vi "RetrieveDefaultRectangleData.vi"(8 "error in (no error)":errorcluster, 10 "Path":path, 11 "Setting Database In":refnum<class "Setting Database.lvclass">) -> (0 "error out":errorcluster, 2 "Rectangle Settings.lvclass":refnum<class "Rectangle Settings.lvclass">, 3 "Setting Database Out":refnum<class "Setting Database.lvclass">)   [LabVIEW 2019, in "Setting Database.lvclass"]
uses:
  Setting Database.lvclass
  Rectangle Settings/Rectangle Settings.lvclass
  Setting Database.lvclass/Setting Database.ctl
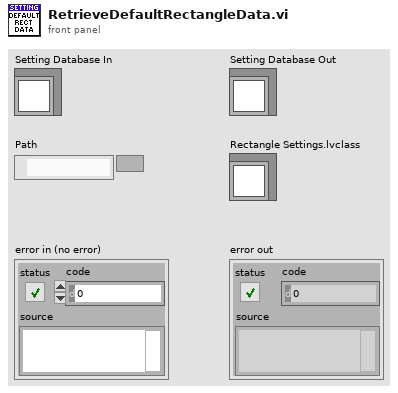
[diagram p1: front panel]
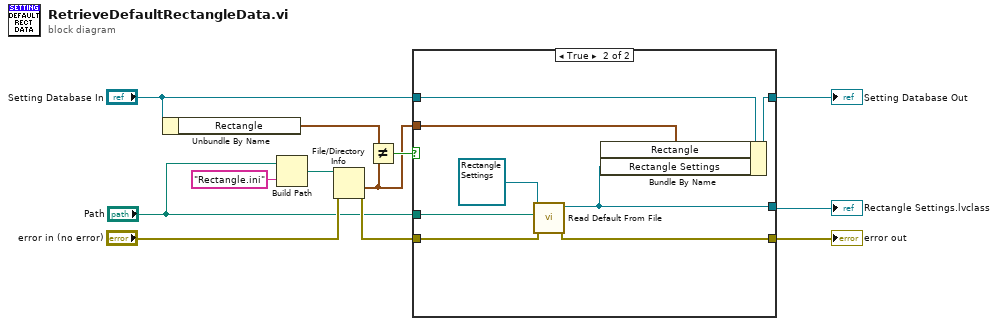
[diagram p0: block diagram]
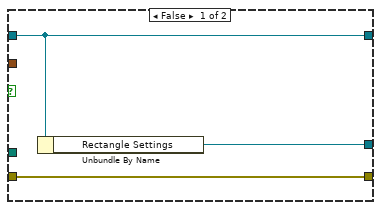
[diagram p2: hidden frame]
diagram:
  n1 = Unbundle By Name("Setting Database In") -> ("Rectangle"=w2:timestamp)
  n2 = Build Path(base path="Path", name or relative path="Rectangle.ini") -> (appended path=w9:path)
  n3 = File/Directory Info(path=w9, error in="error in (no error)") -> (last mod=w1:timestamp, error out=w6:errorcluster)  [unwired: 5 out]
  n4 = Not Equal?(x=w2, y=w1) -> (x != y?=w3:bool)
  n5 = case shown="True" w3 {
    tunnel: [w15 w19] -> w11
    tunnel: "Setting Database In" -> [w14 w22]
    tunnel: [w14 w23] -> w10
    tunnel: w6 -> [w13 w20]
    tunnel: [w13 w21] -> w12
    tunnel: "Path" -> [_ w17]
    tunnel: w1 -> [_ w16]
    frame False {
      n6 = Unbundle By Name(w14) -> ("Rectangle Settings"=w15:refnum<class "Rectangle Settings.lvclass">)
    }
    frame True {
      n7 = call-dynamic "Read Default From File.vi"("error in (no error)"=w20, "Path"=w17, "Rectangle Settings in"=refnum<class "Rectangle Settings.lvclass"> refnum) -> ("error out"=w21:errorcluster, "Rectangle Settings out"=w19:refnum<class "Rectangle Settings.lvclass">)  [unwired: 7 in]
      n8 = Bundle By Name(cluster=w22, "Rectangle"=w16, "Rectangle Settings"=w19) -> (w23:refnum<class "Setting Database.lvclass">)
    }
  }
  "error out" <- w12
  "Rectangle Settings.lvclass" <- w11
  "Setting Database Out" <- w10
